vi "ResetControllerEng.vi"() -> (0 "Error":bool)   [LabVIEW 2014]
panel:
  out "Utility Board":bool
  in  "OK":bool
  in  "Apply":bool
  in  "Close":bool
  in  "Utility Code File":path=path "C:/AzCam/AzCamServer/systems/soguiders/util2.lod" caption="Utility DSP Code File"
  in  "Timing Code File":path=path "C:/AzCam/AzCamServer/systems/soguiders/90guider.lod" caption="Timing DSP Code File"
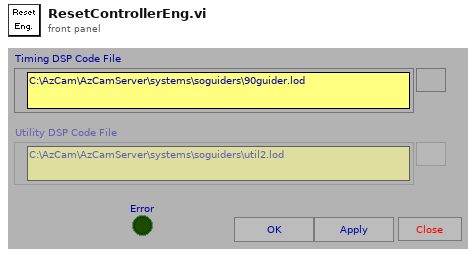
[diagram p1: front panel]
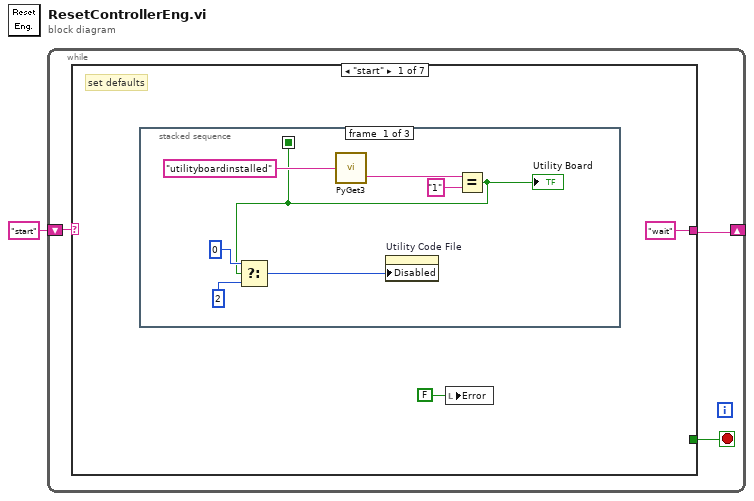
[diagram p0: block diagram]
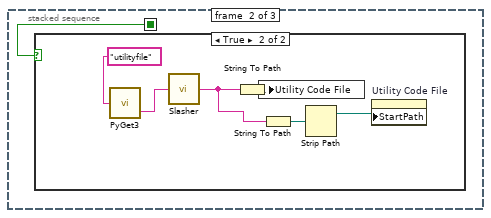
[diagram p2: hidden frame]
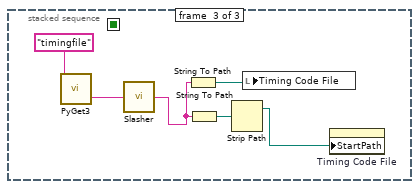
[diagram p4: hidden frame]
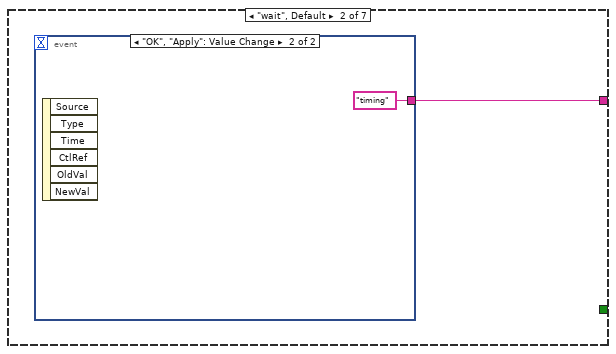
[diagram p5: hidden frame]
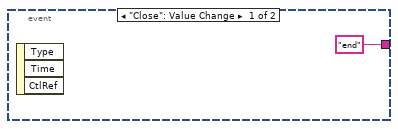
[diagram p6: hidden frame]
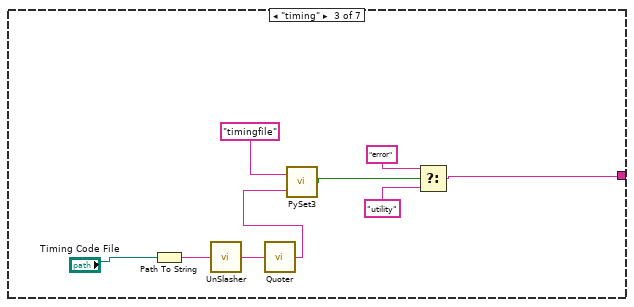
[diagram p7: hidden frame]
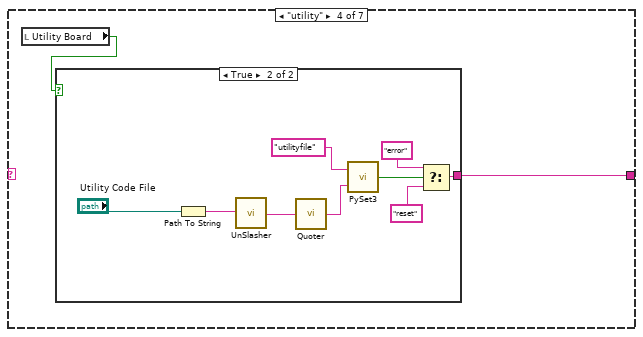
[diagram p8: hidden frame]
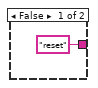
[diagram p9: hidden frame]
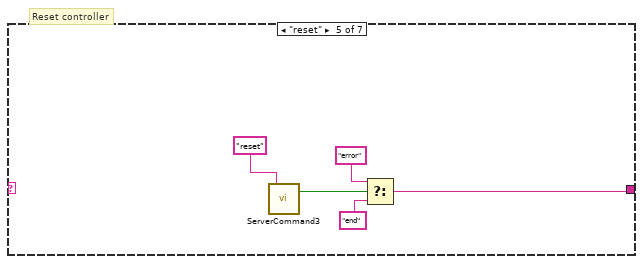
[diagram p10: hidden frame]
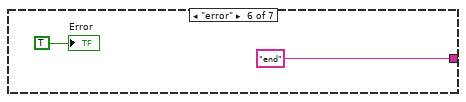
[diagram p11: hidden frame]
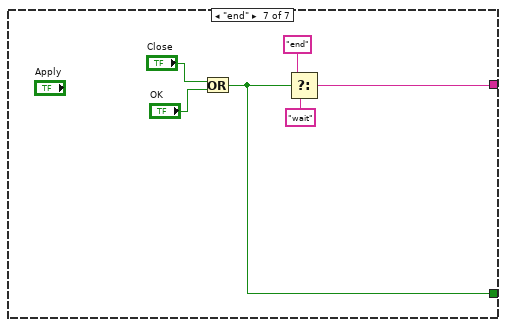
[diagram p12: hidden frame]
diagram:
  n1 = while {
    shift-right: [w2] -> _
    shift-left: "start" -> [w3]
    stop <- w4 stop-if-true
    n2 = case shown="\"start\"" w3 {
      tunnel: [_ _ _ _ _ _ w58] -> w4
      tunnel: ["wait" ("Error String") w27 w36 w40 w53 "end" ("Error String") w61] -> w2
      frame "start" {
        # "set defaults"
        n3 = stacked-sequence {
          seq-local: [w7 _ _] -> [_ w14 _]
          frame #0 {
            n4 = call "PyGet3.vi"("Attribute"="utilityboardinstalled") -> ("Reply"=w9:string)  [unwired: 1 out]
            n5 = Equal?(x=w9, y="1") -> (x = y?=w7:bool)
            "Utility Board" <- w7
            n6 = Select(t=0, s=w7, f=2) -> (s? t:f=w11:i32)
            n7 = property on="Utility Code File" class="Path"("Disabled"=w11) -> ()  [unwired: 2 in, 2 out]
          }
          frame #1 {
            n8 = case shown="True" w14 {
              frame False {
              }
              frame True {
                n9 = call "PyGet3.vi"("Attribute"="utilityfile") -> ("Reply"=w19:string)  [unwired: 1 out]
                n10 = call "Slasher.vi"("String In"=w19) -> ("String Out"=w20:string)
                n11 = String To Path(string=w20) -> (path=w16:path)
                n12 = local write "Utility Code File"(w16) -> ()
                n13 = String To Path(string=w20) -> (path=w18:path)
                n14 = Strip Path(path=w18) -> (stripped path=w17:path)  [unwired: 1 out]
                n15 = property on="Utility Code File" class="Path"("StartPath"=w17) -> ()  [unwired: 2 in, 2 out]
              }
            }
          }
          frame #2 {
            n16 = call "PyGet3.vi"("Attribute"="timingfile") -> ("Reply"=w25:string)  [unwired: 1 out]
            n17 = call "Slasher.vi"("String In"=w25) -> ("String Out"=w26:string)
            n18 = String To Path(string=w26) -> (path=w22:path)
            n19 = String To Path(string=w26) -> (path=w23:path)
            n20 = Strip Path(path=w23) -> (stripped path=w24:path)  [unwired: 1 out]
            n21 = local write "Timing Code File"(w22) -> ()
            n22 = property on="Timing Code File" class="Path"("StartPath"=w24) -> ()  [unwired: 2 in, 2 out]
          }
        }
        n23 = local write "Error"(FALSE ("Error")) -> ()
      }
      frame "wait", Default {
        n24 = event shown="[1] \"OK\", \"Apply\": Value Change" {
          selector: _ -> [_ _]
          dyn-events: _ -> [_ _]
          timeout: _ -> [_ _]
          tunnel: ["end" "timing"] -> w27
          event "Close": Value Change {
            n25 = event-data() -> ()  [unwired: 1 in, 3 out]
          }
          event "OK", "Apply": Value Change {
            n26 = event-data() -> ()  [unwired: 1 in, 6 out]
          }
        }
      }
      frame "timing" {
        # "Init Timing Card"
        n27 = Path To String(path="Timing Code File") -> (string=w34:string)
        n28 = call "UnSlasher.vi"("String In"=w34) -> ("String Out"=w31:string)
        n29 = call "Quoter.vi"("String In"=w31) -> ("String Out"=w30:string)
        n30 = call "PySet3.vi"("Value"=w30, "Attribute"="timingfile" ("Command")) -> ("Error"=w33:bool)
        n31 = Select(t="error" ("Error String"), s=w33, f="utility" ("Error String")) -> (s? t:f=w36:string)
      }
      frame "utility" {
        # "Init Utility Card"
        n32 = local read "Utility Board"() -> (w39:bool)
        n33 = case shown="True" w39 {
          tunnel: ["reset" ("Error String") w50] -> w40
          frame False {
          }
          frame True {
            n34 = Path To String(path="Utility Code File") -> (string=w46:string)
            n35 = call "UnSlasher.vi"("String In"=w46) -> ("String Out"=w43:string)
            n36 = call "Quoter.vi"("String In"=w43) -> ("String Out"=w42:string)
            n37 = call "PySet3.vi"("Value"=w42, "Attribute"="utilityfile" ("Command")) -> ("Error"=w45:bool)
            n38 = Select(t="error" ("Error String"), s=w45, f="reset" ("Error String")) -> (s? t:f=w50:string)
          }
        }
      }
      frame "reset" {
        # "Reset controller"
        n39 = call "ServerCommand3.vi"("Command"="reset") -> ("Error"=w51:bool)  [unwired: 1 out]
        n40 = Select(t="error" ("Error String"), s=w51, f="end" ("Error String")) -> (s? t:f=w53:string)
      }
      frame "error" {
        "Error" <- TRUE ("Error")
      }
      frame "end" {
        n41 = Or(x="Close", y="OK") -> (x .or. y?=w58:bool)
        n42 = Select(t="end", s=w58, f="wait") -> (s? t:f=w61:string)
      }
    }
  }
